vi "PostCalibration.vi"(8 "error in (no error)":errorcluster, 11 "ByteGSWebAPI-V0 in":refnum<class "ByteGSWebAPI-V0.lvclass">) -> (0 "error out":errorcluster, 3 "ByteGSWebAPI-V0 out":refnum<class "ByteGSWebAPI-V0.lvclass">)   [LabVIEW 2019, in "ByteGSWebAPI.lvlib" / "ByteGSWebAPI-V0.lvclass"]
uses:
  ByteGSWebAPI-V0.lvclass
  42e497da-5ad5-43d4-ba9e-122ef82835be.vi
  Cntrls/SingleCalibration.ctl
panel:
  out "body":string
  out "headers":string
  in  "Calibration":T1
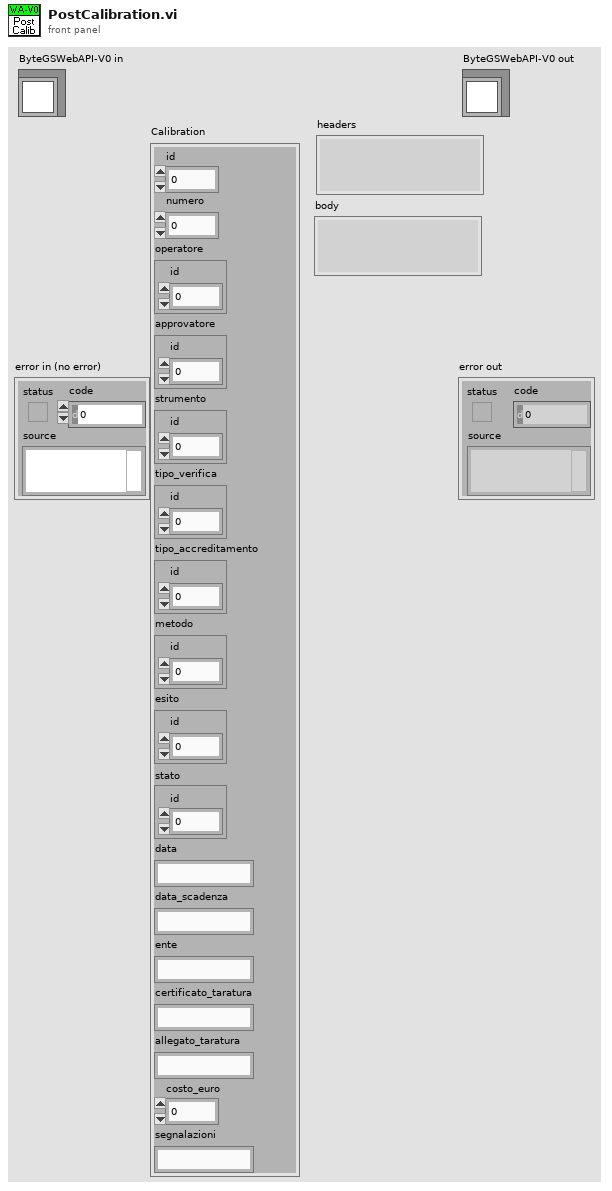
[diagram p1: front panel]
types:
  T1 = typedef "ByteGSWebAPI.lvlib/ByteGSWebAPI-V0.lvclass/SingleCalibration.ctl" = cluster{"id":i32, "numero":i32, "operatore":cluster{"id":i32}, "approvatore":cluster{"id":i32}, "strumento":cluster{"id":i32}, "tipo_verifica":cluster{"id":i32}, "tipo_accreditamento":cluster{"id":i32}, "metodo":cluster{"id":i32}, "esito":cluster{"id":i32}, "stato":cluster{"id":i32}, "data":string, "data_scadenza":string, "ente":string, "certificato_taratura":string, "allegato_taratura":string, "costo_euro":dbl, "segnalazioni":string}
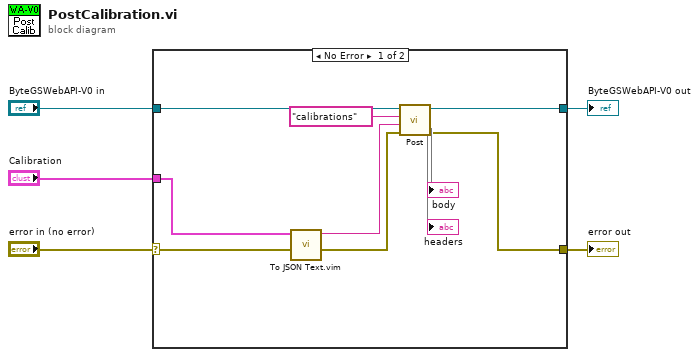
[diagram p0: block diagram]
diagram:
  n1 = case shown="No Error" "error in (no error)" {
    selector: "error in (no error)" -> [w12 w17]
    tunnel: [w6 w17] -> w4
    tunnel: [w15 w16] -> w2
    tunnel: "ByteGSWebAPI-V0 in" -> [w14 w16]
    tunnel: "Calibration" -> [w11 _]
    frame No Error {
      n2 = call "To JSON Text.vim"("error in (no error)"=w12, "Anything"=w11) -> ("error out"=w7:errorcluster, "<JSON>"=w10:string)  [unwired: 8 in]
      n3 = call "Post.vi"("error in (no error)"=w7, "Buffer"=w10, "Request"="calibrations", "ByteGSWebAPI-V0 in"=w14) -> ("error out"=w6:errorcluster, "ByteGSWebAPI-V0 out"=w15:refnum<class "ByteGSWebAPI-V0.lvclass">, 4:→"body", 6:→"headers")  [unwired: 2 in, 2 out]
    }
    frame Error {
    }
  }
  "error out" <- w4
  "ByteGSWebAPI-V0 out" <- w2
